vi "CalcularArea.vi"(8 "error in":errorcluster, 11 "object in":refnum<class "Triangulo.lvclass">) -> (0 "error out":errorcluster, 2 "Area":dbl, 3 "object out":refnum<class "Triangulo.lvclass">)   [LabVIEW 2024, in "Triangulo.lvclass"]
uses:
  Triangulo.lvclass
  Triangulo.lvclass/Triangulo.ctl
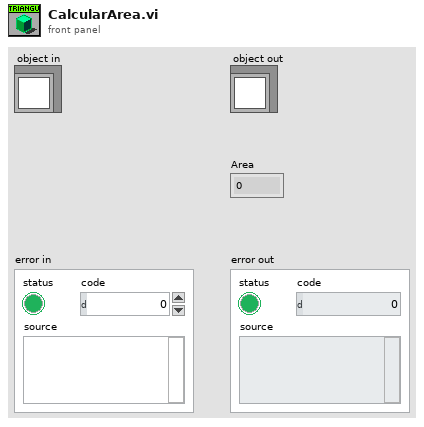
[diagram p1: front panel]
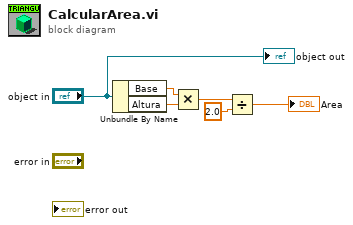
[diagram p0: block diagram]
diagram:
  n1 = Unbundle By Name("object in") -> ("Base"=w5:dbl, "Altura"=w4:dbl)
  n2 = Multiply(x=w5, y=w4) -> (x*y=w3:dbl)
  n3 = Divide(x=w3, y=2.0) -> (x/y=→"Area":dbl)
  "object out" <- "object in"
